vi "Comparador.vi"() -> ()   [LabVIEW 2018]
panel:
  out "A>B":bool
  out "B":bool[](array[boolean])
  out "A":bool[](array[boolean])
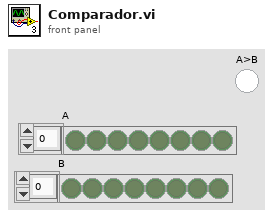
[diagram p1: front panel]
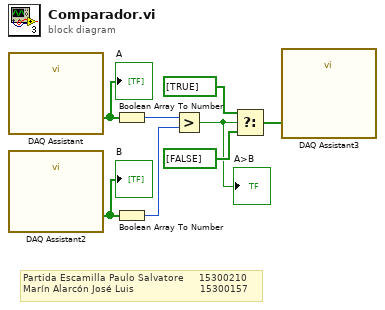
[diagram p0: block diagram]
diagram:
  # "Partida Escamilla Paulo Salvatore     15300210\nMarín Alarcón José Luis                      15300157"
  n1 = call "DAQ Assistant"() -> ("data"=w8:bool[])  [unwired: 17 in, 2 out]
  "A" <- w8
  n2 = call "DAQ Assistant2"() -> ("data"=w7:bool[])  [unwired: 17 in, 2 out]
  "B" <- w7
  n3 = Boolean Array To Number(Boolean array=w8) -> (number=w6:u32)
  n4 = Boolean Array To Number(Boolean array=w7) -> (number=w5:u32)
  n5 = Greater?(x=w6, y=w5) -> (0:w1:bool)
  "A>B" <- w1
  n6 = Select(t=bool[] [TRUE] ("data"), s=w1, f=bool[] [FALSE] ("data")) -> (s? t:f=w2:bool[])
  n7 = call "DAQ Assistant3"("data"=w2) -> ()  [unwired: 17 in, 2 out]
